vi "Read Serialized.vi"(8 "error in (no error)":errorcluster, 11 "ToneCloud in":refnum<class "Tone Cloud.lvclass">) -> (0 "error out":errorcluster, 2 "Serialized":T1, 3 "ToneCloud out":refnum<class "Tone Cloud.lvclass">)   [LabVIEW 2020, in "Tone Cloud.lvclass"]
uses:
  Tone Cloud.lvclass
  Serialized.ctl
  Spacing.ctl
  Level Mode.ctl
  Tone Cloud.lvclass/Tone Cloud.ctl
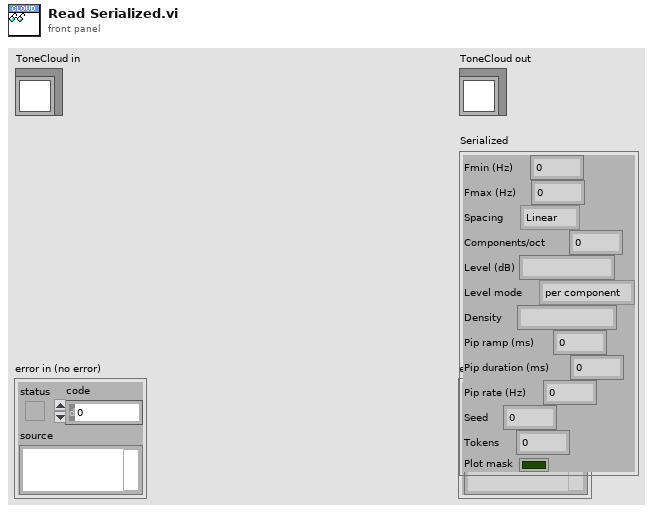
[diagram p1: front panel]
types:
  T1 = typedef "Tone Cloud.lvclass/Serialized.ctl" = cluster{"Fmin (Hz)":dbl, "Fmax (Hz)":dbl, "Spacing":T2, "Components/oct":dbl, "Level (dB)":string, "Level mode":T3, "Density":string, "Pip ramp (ms)":dbl, "Pip duration (ms)":dbl, "Pip rate (Hz)":dbl, "Seed":i32, "Tokens":i32, "Plot mask":bool}
  T2 = typedef "Tone Cloud.lvclass/Spacing.ctl" = enum16{"Linear", "Log"}
  T3 = typedef "Tone Cloud.lvclass/Level Mode.ctl" = enum16{"per component", "total rms"}
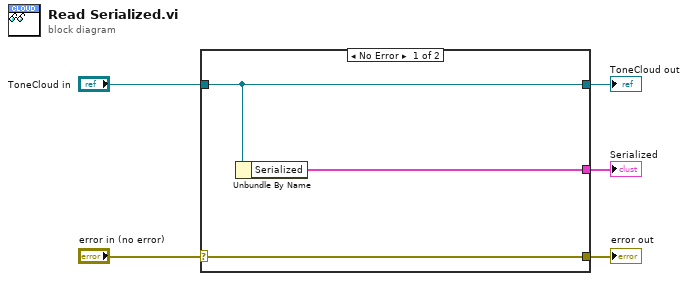
[diagram p0: block diagram]
diagram:
  n1 = case shown="No Error" "error in (no error)" {
    selector: "error in (no error)" -> [w8 w9]
    tunnel: [w8 w9] -> w4
    tunnel: [w7 w10] -> w2
    tunnel: "ToneCloud in" -> [w7 w10]
    tunnel: [w6 _] -> w1
    frame No Error {
      n2 = Unbundle By Name(w7) -> ("Serialized"=w6:T1)
    }
    frame Error {
    }
  }
  "error out" <- w4
  "ToneCloud out" <- w2
  "Serialized" <- w1
